vi "Kalman filter - test loop.vi"() -> ()   [LabVIEW 2013]
uses:
  <vilib>/Utility/file.llb/Read From Spreadsheet File (I64).vi
panel:
  in  "Constants":T1={"Q_Angle"=0.001, "Q_Bias"=0.003, "R_measure"=0.03}
  out "Waveform Chart":dbl(graph)
  in  "file path (dialog if empty)":path=path "C:/Documents and Settings/Marcin Twardak/Moje dokumenty/GitHub/quadro-controller/Wersja do własnego programu/STM32F100/dane_akc.txt"
  # "Process noise variance\nfor the accelerometer"
  # "Process noise variance\nfor the gyro bias"
  # "Measurement noise variance - \nthis is actually the variance \nof the measurement noise"
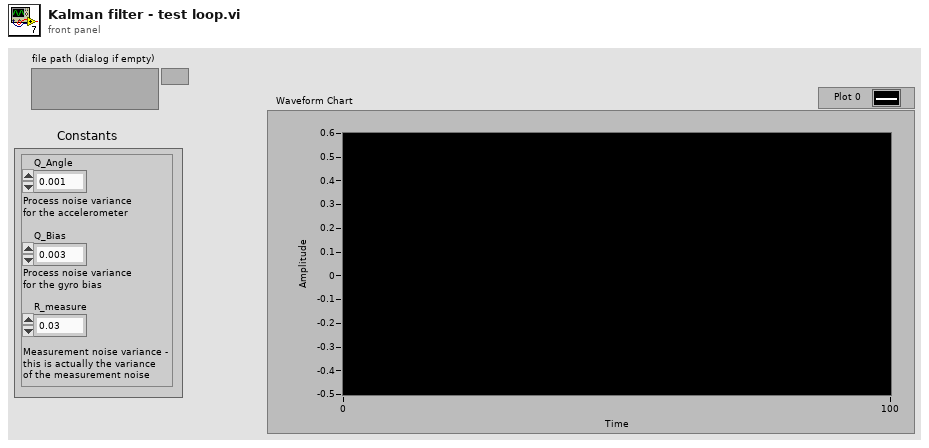
[diagram p1: front panel]
types:
  T1 = cluster{"Q_Angle":dbl, "Q_Bias":dbl, "R_measure":dbl}
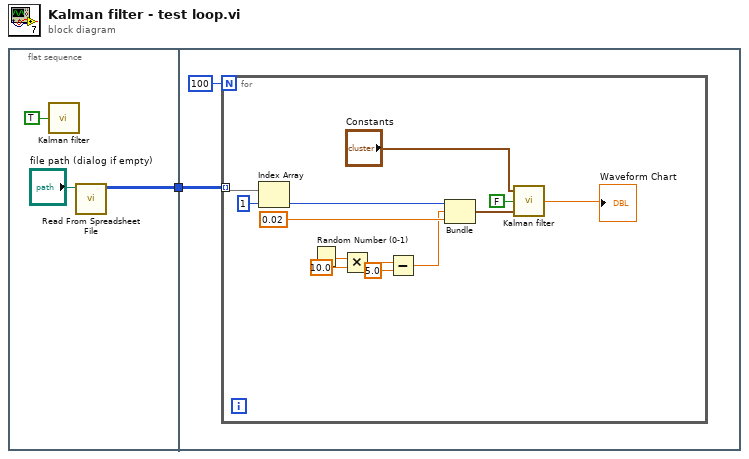
[diagram p0: block diagram]
diagram:
  n1 = flat-sequence {
    tunnel: [w2] -> w1
    tunnel: w1 -> [w5]
    frame #0 {
      n2 = call "Kalman filter.vi"("Reset"=TRUE) -> ()  [unwired: 2 in, 1 out]
      n3 = call-poly <vilib>:"Read From Spreadsheet File.vi"("file path (dialog if empty)"="file path (dialog if empty)") -> ("all rows"=w2:i64[][])  [unwired: 6 in, 4 out]
    }
    frame #1 {
      n4 = for {
        N: 100 -> [_]
        tunnel: w5 -> [w19] mode=indexing
        n5 = Index Array(array=w19, index=1) -> (element=w17:i64)
        n6 = Random Number (0-1)() -> (number: 0 to 1=w15:dbl)
        n7 = Multiply(x=w15, y=10.0) -> (x*y=w13:dbl)
        n8 = Subtract(x=w13, y=5.0) -> (x-y=w11:dbl)
        n9 = Bundle(w17, w11, 0.02) -> (w10:cluster{i64, dbl, dbl})  [unwired: 1 in]
        n10 = call "Kalman filter.vi"("New data"=w10, "Reset"=FALSE, "Constants"="Constants") -> ("Angle out"=→"Waveform Chart":dbl)
      }
    }
  }
